vi "Garmin Parse RMC.vi"(8 "RMC":T1 {"Long" format="%.6f"; "Course" format="%.2f"; "Speed" format="%.2f"; "Lat" format="%.6f"}, 9 "Input":string) -> (1 "OK":bool, 2 "RMC":T1 {"Long" format="%.6f"; "Course" format="%.2f"; "Speed" format="%.2f"; "Lat" format="%.6f"}, 3 "Raw RMC":T2)   [LabVIEW 2015]
uses:
  RMC.ctl
  Raw RMC.ctl
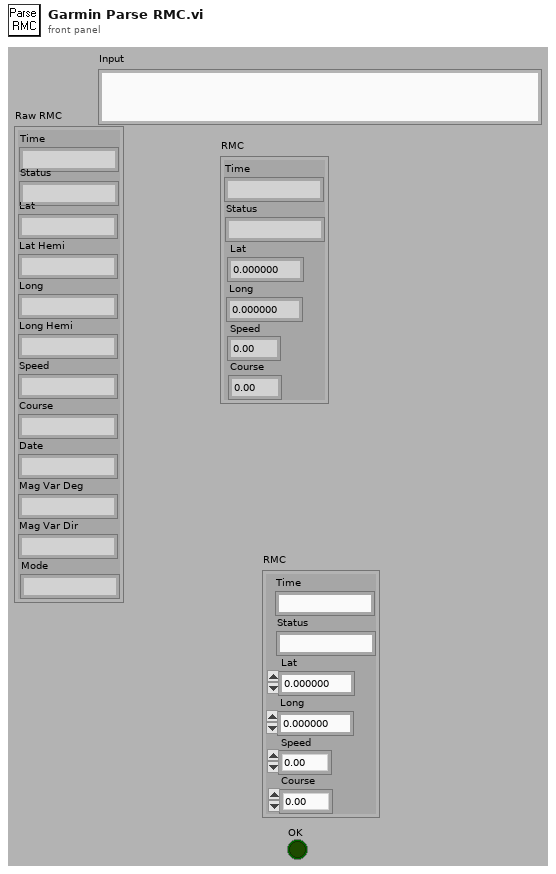
[diagram p1: front panel]
types:
  T1 = typedef "RMC.ctl" = cluster{"Time":string, "Status":string, "Lat":dbl, "Speed":dbl, "Course":dbl, "Long":dbl}
  T2 = typedef "Raw RMC.ctl" = cluster{"Time":string, "Status":string, "Lat":string, "Lat Hemi":string, "Long":string, "Long Hemi":string, "Speed":string, "Course":string, "Date":string, "Mag Var Deg":string, "Mag Var Dir":string, "Mode":string}
  T3 = cluster{"[0]":string, "[1]":string, "[2]":string, "[3]":string, "[4]":string, "[5]":string, "[6]":string, "[7]":string, "[8]":string, "[9]":string, "[10]":string, "[11]":string}
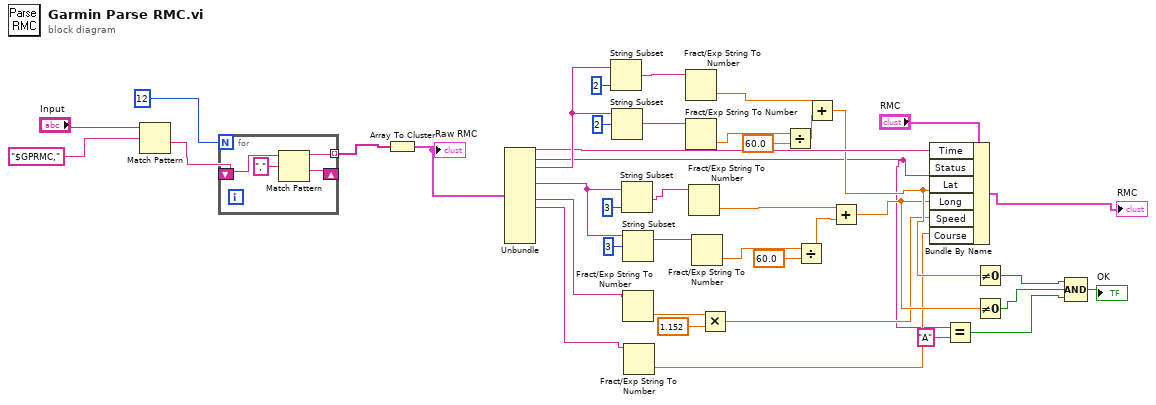
[diagram p0: block diagram]
diagram:
  n1 = Match Pattern(string="Input", regular expression="$GPRMC,") -> (after substring=w40:string)  [unwired: 1 in, 3 out]
  n2 = for {
    N: 12 ("Numeric") -> [_]
    shift-right: [w44] -> _
    shift-left: w40 -> [w42]
    tunnel: [w43] -> w38 mode=indexing
    n3 = Match Pattern(string=w42, regular expression=",") -> (before substring=w43:string, after substring=w44:string)  [unwired: 1 in, 2 out]
  }
  n4 = Array To Cluster(array=w38) -> (cluster=w37:T3)
  "Raw RMC" <- w37
  n5 = Unbundle(w37) -> ("[0]"=w19:string, "[1]"=w3:string, "[2]"=w34:string, "[4]"=w30:string, "[6]"=w25:string, "[7]"=w24:string)  [unwired: 6 out]
  n6 = String Subset(string=w34, length (rest)=2 ("length (rest)")) -> (substring=w26:string)  [unwired: 1 in]
  n7 = String Subset(string=w34, offset (0)=2) -> (substring=w27:string)  [unwired: 1 in]
  n8 = String Subset(string=w30, length (rest)=3 ("length (rest)")) -> (substring=w28:string)  [unwired: 1 in]
  n9 = String Subset(string=w30, offset (0)=3) -> (substring=w29:string)  [unwired: 1 in]
  n10 = Fract/Exp String To Number(string=w25) -> (number=w21:dbl)  [unwired: 3 in, 1 out]
  n11 = Fract/Exp String To Number(string=w24) -> (number=w7:dbl)  [unwired: 3 in, 1 out]
  n12 = Fract/Exp String To Number(string=w26) -> (number=w22:dbl)  [unwired: 3 in, 1 out]
  n13 = Fract/Exp String To Number(string=w27) -> (number=w16:dbl)  [unwired: 3 in, 1 out]
  n14 = Fract/Exp String To Number(string=w28) -> (number=w23:dbl)  [unwired: 3 in, 1 out]
  n15 = Fract/Exp String To Number(string=w29) -> (number=w14:dbl)  [unwired: 3 in, 1 out]
  n16 = Multiply(x=w21, y=1.152) -> (x*y=w8:dbl)
  n17 = Divide(x=w16, y=60.0) -> (x/y=w18:dbl)
  n18 = Divide(x=w14, y=60.0) -> (x/y=w13:dbl)
  n19 = Add(x=w22, y=w18) -> (x+y=w10:dbl)
  n20 = Add(x=w23, y=w13) -> (x+y=w9:dbl)
  n21 = Bundle By Name(cluster="RMC", "Time"=w19, "Status"=w3, "Lat"=w10, "Long"=w9, "Speed"=w8, "Course"=w7) -> (→"RMC":T1)
  n22 = Equal?(x=w3, y="A") -> (x = y?=w1:bool)
  n23 = Not Equal To 0?(x=w10) -> (x != 0?=w6:bool)
  n24 = Not Equal To 0?(x=w9) -> (x != 0?=w5:bool)
  n25 = Compound Arithmetic op=AND(w6, w5, w1) -> (→"OK":bool)
